vi "PCO_InitLensControl.vi"(8 "error in (no error)":errorcluster {"code" format="%x"}, 11 "ph":u64) -> (0 "error out":errorcluster {"code" format="%x"}, 1 "hLens out":u64, 2 "ErrorMessage":i32 format="%x", 3 "ph out":u64)   [LabVIEW 2020, in "SDK.lvlib" / "LensControl.lvlib"]
doc: "<b>Description:</b>\nInitializes a new lens control object when phLensControl is NULL and returns the handle to the internal structures.\nAlso reinitializes an already existing lens control object when called with a valid phLensControl.\nE.g. when the lens is changed in front of the Birger ring the lens functions will return an error as there is no lens for a short time. To reinitialize the lens after re-plug, call PCO_InitLensControl with a previously created and valid phLensControl. You can use a windows timer function in order to call the init function till it returns without error. Processing can be continued normally after successful re-initialization.\nAs the interface is a serial port the initialization takes some time.\nIt is mandatory to call PCO_CloseLensControl or PCO_CleanupLensControl during shutdown of the application.\n\n<b>Supported camera type:</b>\npco.edge CLHS, pco.dimax cs\n\n<b>Descriptor dependency:</b>\ndwGeneralCapsDESC1: GENERALCAPS1_USER_INTERFACE"
uses:
  LensControl.lvlib
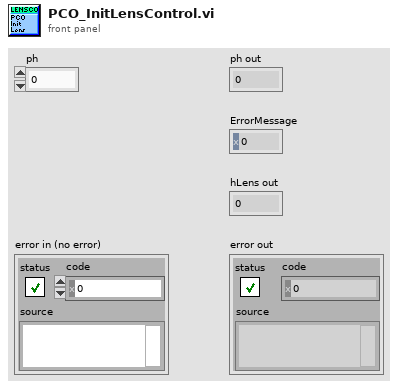
[diagram p1: front panel]
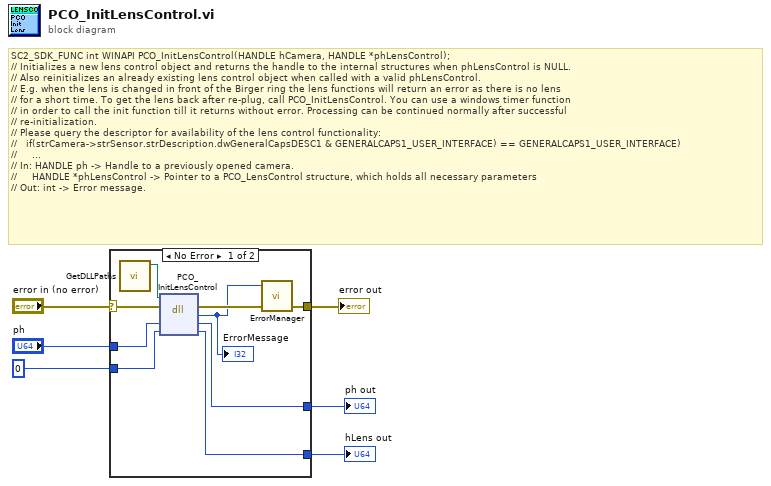
[diagram p0: block diagram]
diagram:
  # "SC2_SDK_FUNC int WINAPI PCO_InitLensControl(HANDLE hCamera, HANDLE *phLensControl);\n// Initializes a new lens control object and returns the handle to the internal structures when phLensControl is NULL.\n// Also reinitializes an already existing lens control object when called with a valid phLensControl.\n// E.g. when the lens is changed in front of the Birger ring the lens functions will return an error as there is no lens \n// for a short time. To get the lens back after re-plug, call PCO_InitLensControl. You can use a windows timer function\n// in order to call the init function till it returns without error. Processing can be continued normally after successful\n// re-initialization.\n// Please query the descriptor for availability of the lens control functionality:\n//   if(strCamera->strSensor.strDescription.dwGeneralCapsDESC1 & GENERALCAPS1_USER_INTERFACE) == GENERALCAPS1_USER_INTERFACE)\n//     ...\n// In: HANDLE ph -> Handle to a previously opened camera.\n//     HANDLE *phLensControl -> Pointer to a PCO_LensControl structure, which holds all necessary parameters\n// Out: int -> Error message."
  n1 = case shown="No Error" "error in (no error)" {
    selector: "error in (no error)" -> [w11 w16]
    tunnel: "ph" -> [w15 w18]
    tunnel: [w14 w18] -> w5
    tunnel: u64 0 ("hLens") -> [w13 w17]
    tunnel: [w12 w17] -> w3
    tunnel: [w10 w16] -> w2
    frame No Error {
      n2 = call "GetDLLPaths.vi"() -> ("SC2_Cam_Path"=w7:path)  [unwired: 9 in, 2 out]
      n3 = dll-call lib="?" fn="PCO_InitLensControl"(path in=w7, error in=w11, "ph"=w15, "hLens"=w13) -> (error out=w9:errorcluster, "return type"=w8:i32, "ph"=w14:u64, "hLens"=w12:u64)  [unwired: 1 in, 1 out]
      "ErrorMessage" <- w8
      n4 = call "ErrorManager.vi"("error in (no error)"=w9, "error code"=w8) -> ("error out"=w10:errorcluster)  [unwired: 3 in]
    }
    frame Error {
    }
  }
  "ph out" <- w5
  "hLens out" <- w3
  "error out" <- w2
